vi "auto avance ralentir.vi"(9 "vitesse gauche":dbl, 10 "temps":dbl, 11 "temps de changement de direction":dbl) -> ()   [LabVIEW 2015]
uses:
  <vilib>/Rock Robotics/WPI/Solenoid/WPI_SolenoidValue.ctl
  <vilib>/Rock Robotics/WPI/Solenoid/WPI_SolenoidSetEnum.vi
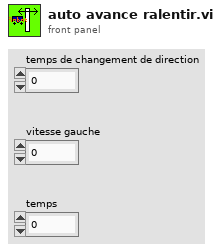
[diagram p1: front panel]
types:
  T1 = typedef "WPI_SolenoidValue.ctl" = enum16{"Off", "On", "Forward", "Reverse"}
  T2 = typedef "WPI_ServoDeviceRef.ctl" = cluster{"DeviceStatus":errorcluster, "PWM Channel":T3, "DeadBand":T4}
  T3 = typedef "FPGA_DIOPWMChannel.ctl" = enum8{"PWM 0", "PWM 1", "PWM 2", "PWM 3", "PWM 4", "PWM 5", "PWM 6", "PWM 7", "PWM 8", "PWM 9", "PWM MXP 0", "PWM MXP 1", "PWM MXP 2", "PWM MXP 3", "PWM MXP 4", "PWM MXP 5", "PWM MXP 6", "PWM MXP 7", "PWM MXP 8", "PWM MXP 9", "Invalid"}
  T4 = typedef "WPI_PWMDeadband.ctl" = cluster{"Name":string, "maxPositivePwm":i32, "minPositivePwm":i32, "centerPwm":i32, "maxNegativePwm":i32, "minNegativePwm":i32, "angularRange":u16}
  T5 = typedef "WPI_SolenoidDevRef.ctl" = cluster{"DevStatus":errorcluster, "Pneumatics Control Module":u8, "Forward Solenoid Channel":T6, "Reverse Solenoid Channel":T6}
  T6 = typedef "WPI_SolenoidChannel.ctl" = enum8{"Solenoid 0", "Solenoid 1", "Solenoid 2", "Solenoid 3", "Solenoid 4", "Solenoid 5", "Solenoid 6", "Solenoid 7", "Invalid"}
  T7 = typedef "WPI_EncoderDevRef.ctl" = cluster{"DevStatus":errorcluster, "EncoderIndex":T8, "CounterIndex":T9, "DistancePerCount":dbl, "Decoding Type":T10}
  T8 = typedef "FPGA_EncoderIdx.ctl" = enum8{"Enc 0", "Enc 1", "Enc 2", "Enc 3", "Enc 4", "Enc 5", "Enc 6", "Enc 7", "Invalid"}
  T9 = typedef "FPGA_CounterCtrSystemIndex.ctl" = enum8{"Ctr 0", "Ctr 1", "Ctr 2", "Ctr 3", "Ctr 4", "Ctr 5", "Ctr 6", "Ctr 7", "Invalid"}
  T10 = typedef "WPI_EncoderType.ctl" = enum16{"1x", "2x", "4x"}
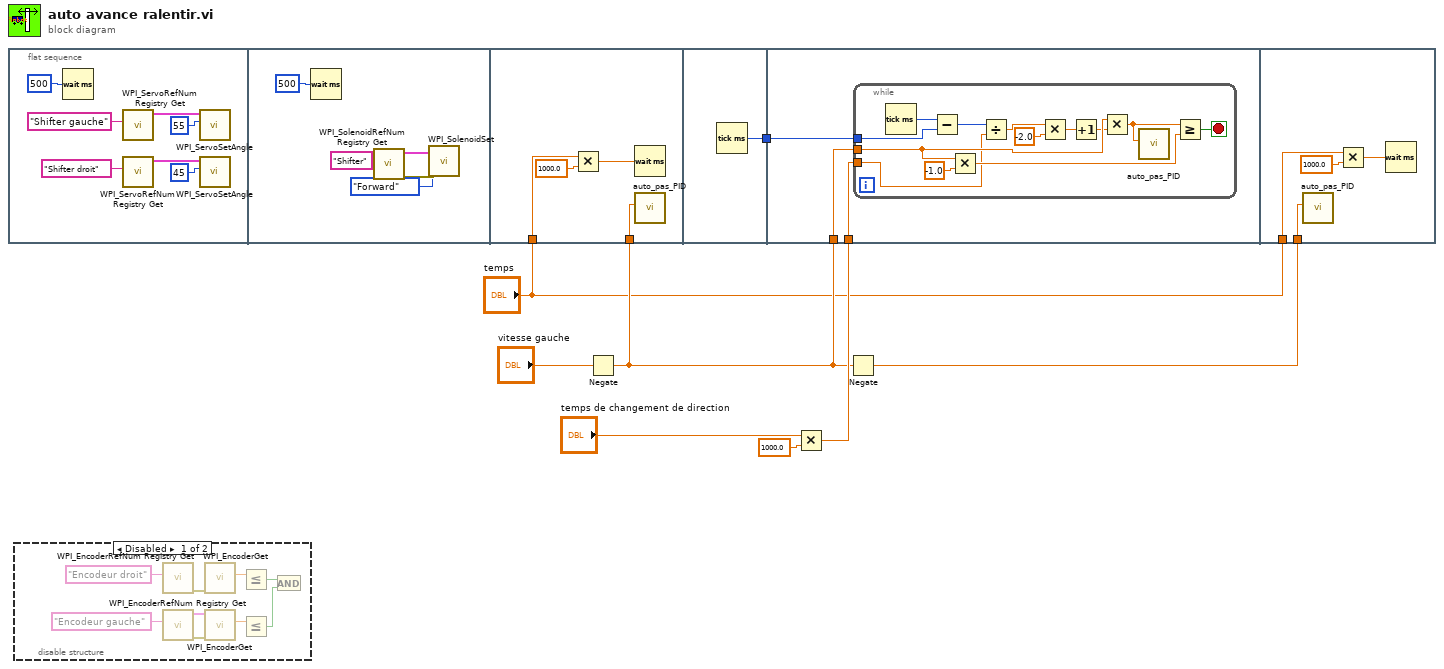
[diagram p0: block diagram]
diagram:
  n1 = flat-sequence {
    tunnel: w3 -> [w24]
    tunnel: "temps" -> [w22]
    tunnel: [w25] -> w8
    tunnel: w8 -> [w28]
    tunnel: w3 -> [w27]
    tunnel: w5 -> [w26]
    tunnel: w2 -> [w45]
    tunnel: "temps" -> [w42]
    frame #0 {
      n2 = Wait (ms)(milliseconds to wait=u32 500) -> ()  [unwired: 1 out]
      n3 = call <vilib>:"WPI_ServoRefNum Registry Get.vi"("refnum name"="Shifter gauche") -> ("ServoDeviceRef"=w14:T2)  [unwired: 9 in, 1 out]
      n4 = call <vilib>:"WPI_ServoRefNum Registry Get.vi"("refnum name"="Shifter droit") -> ("ServoDeviceRef"=w15:T2)  [unwired: 9 in, 1 out]
      n5 = call <vilib>:"WPI_ServoSetAngle.vi"("Angle"=55, "ServoDeviceRef"=w14) -> ()  [unwired: 8 in, 2 out]
      n6 = call <vilib>:"WPI_ServoSetAngle.vi"("Angle"=45, "ServoDeviceRef"=w15) -> ()  [unwired: 8 in, 2 out]
    }
    frame #1 {
      n7 = Wait (ms)(milliseconds to wait=u32 500) -> ()  [unwired: 1 out]
      n8 = call <vilib>:"WPI_SolenoidRefNum Registry Get.vi"("refnum name"="Shifter") -> ("error out"=w18:errorcluster, "SolenoidDevRef"=w17:T5)  [unwired: 9 in]
      n9 = call-poly <vilib>:"WPI_SolenoidSet.vi"("error in (no error)"=w18, "Value"=WPI_SolenoidValue."Forward", "SolenoidDevRef"=w17) -> ()  [unwired: 7 in, 2 out]
    }
    frame #2 {
      n10 = Multiply(x=w22, y=1000.0) -> (x*y=w21:dbl)
      n11 = Wait (ms)(milliseconds to wait=w21) -> ()  [unwired: 1 out]
      n12 = call "auto_pas_PID.vi"("vitesse voulu"=w24) -> ()  [unwired: 11 in]
    }
    frame #3 {
      n13 = Tick Count (ms)() -> (millisecond timer value=w25:u32)
    }
    frame #4 {
      n14 = while {
        tunnel: w28 -> [w32]
        tunnel: w27 -> [w40]
        tunnel: w26 -> [w38]
        stop <- w29 stop-if-true
        n15 = Tick Count (ms)() -> (millisecond timer value=w31:u32)
        n16 = Subtract(x=w31, y=w32) -> (x-y=w37:u32)
        n17 = Multiply(x=w40, y=-1.0) -> (x*y=w39:dbl)
        n18 = Divide(x=w37, y=w38) -> (x/y=w35:dbl)
        n19 = Multiply(x=w35, y=-2.0) -> (x*y=w34:dbl)
        n20 = Increment(x=w34) -> (x+1=w33:dbl)
        n21 = Multiply(x=w40, y=w33) -> (x*y=w30:dbl)
        n22 = call "auto_pas_PID.vi"("vitesse voulu"=w30) -> ()  [unwired: 11 in]
        n23 = Greater Or Equal?(x=w30, y=w39) -> (x >= y?=w29:bool)
      }
    }
    frame #5 {
      n24 = call "auto_pas_PID.vi"("vitesse voulu"=w45) -> ()  [unwired: 11 in]
      n25 = Multiply(x=w42, y=1000.0) -> (x*y=w44:dbl)
      n26 = Wait (ms)(milliseconds to wait=w44) -> ()  [unwired: 1 out]
    }
  }
  n27 = disable-structure shown="Disabled" {
    frame Disabled {
      n28 = call <vilib>:"WPI_EncoderRefNum Registry Get.vi"("refnum name"="Encodeur droit") -> ("error out"=w46:errorcluster)  [unwired: 9 in, 1 out]
      n29 = call <vilib>:"WPI_EncoderRefNum Registry Get.vi"("refnum name"="Encodeur gauche") -> ("error out"=w48:errorcluster, "EncoderDevRef"=w49:T7)  [unwired: 9 in]
      n30 = call <vilib>:"WPI_EncoderGet.vi"("error in (no error)"=w46) -> ("Distance"=w51:dbl)  [unwired: 5 in, 5 out]
      n31 = call <vilib>:"WPI_EncoderGet.vi"("error in (no error)"=w48, "EncoderDevRef"=w49) -> ("Distance"=w54:dbl)  [unwired: 4 in, 5 out]
      n32 = Less Or Equal?(x=w51) -> (x <= y?=w52:bool)  [unwired: 1 in]
      n33 = Less Or Equal?(x=w54) -> (x <= y?=w53:bool)  [unwired: 1 in]
      n34 = And(x=w52, y=w53) -> ()  [unwired: 1 out]
    }
    frame Enabled {
    }
  }
  n35 = Negate(x="vitesse gauche") -> (-x=w3:dbl)
  n36 = Multiply(x="temps de changement de direction", y=1000.0) -> (x*y=w5:dbl)
  n37 = Negate(x=w3) -> (-x=w2:dbl)
